vi "toindcluster.vi"(11 "data":T4) -> (1 "B[mT]":dbl, 2 "ROI":T3, 3 "Images":T1)   [LabVIEW 2011]
uses:
  dataTypdef.ctl
  IMAQ Image.ctl
  ROIStartfromCam_typdef.ctl
  analysis_data_typdef.ctl
  MagAnalysis_Online.lvclass
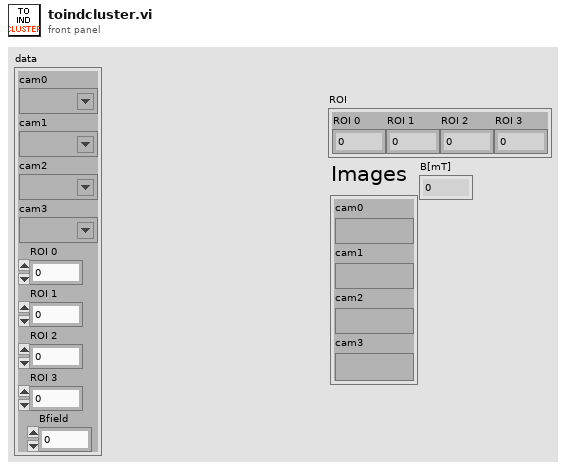
[diagram p1: front panel]
types:
  T1 = typedef "MagAnalysis_Online.lvclass/analysis_data_typdef.ctl" = cluster{"cam0":T2, "cam1":T2, "cam2":T2, "cam3":T2}
  T2 = typedef "IMAQ Image.ctl" = refnum<image>
  T3 = typedef "ROIStartfromCam_typdef.ctl" = cluster{"ROI 0":dbl, "ROI 1":dbl, "ROI 2":dbl, "ROI 3":dbl}
  T4 = typedef "dataTypdef.ctl" = cluster{"cam0":T2, "cam1":T2, "cam2":T2, "cam3":T2, "ROI 0":dbl, "ROI 1":dbl, "ROI 2":dbl, "ROI 3":dbl, "Bfield":dbl}
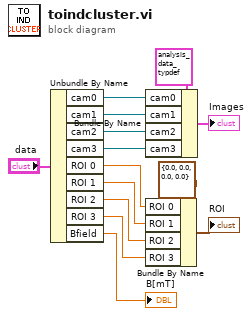
[diagram p0: block diagram]
diagram:
  n1 = Unbundle By Name("data") -> ("cam0"=w12:T2, "cam1"=w11:T2, "cam2"=w10:T2, "cam3"=w9:T2, "ROI 0"=w6:dbl, "ROI 1"=w5:dbl, "ROI 2"=w4:dbl, "ROI 3"=w3:dbl, "Bfield"=→"B[mT]":dbl)
  n2 = Bundle By Name(cluster=T1 {"cam0"=refnum, "cam1"=refnum, "cam2"=refnum, "cam3"=refnum} ("Images 2"), "cam0"=w12, "cam1"=w11, "cam2"=w10, "cam3"=w9) -> (→"Images":T1)
  n3 = Bundle By Name(cluster=T3 {"ROI 0"=0.0, "ROI 1"=0.0, "ROI 2"=0.0, "ROI 3"=0.0} ("ROI"), "ROI 0"=w6, "ROI 1"=w5, "ROI 2"=w4, "ROI 3"=w3) -> (→"ROI":T3)
